vi "Normal Random.vi"(6 "seed":i32=-1, 7 "reset":bool, 9 "std":dbl=1.0, 10 "mean":dbl, 11 "samples":i32=128) -> (0 "error":i32, 3 "normal random data":dbl[](array[numeric]))   [LabVIEW 2024, in "NI_Gmath.lvlib"]
doc: "<p>Generates random values from a variate X, where X describes the selected distribution type. You must <a href=\"nihelplauncher://docs/csh?context=lvcore_lvhowto_selectingdefaultinstpolyvi\">manually select the polymorphic instance</a> to use.</p>"
uses:
  NI_Gmath.lvlib
  NI_AALBase.lvlib
panel:
  # "Normal Random"
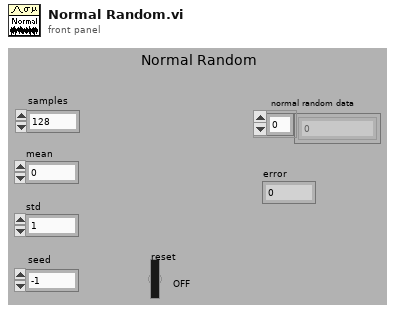
[diagram p1: front panel]
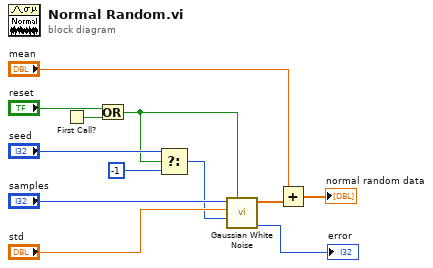
[diagram p0: block diagram]
diagram:
  n1 = First Call?() -> (First Call?: T/F=w12:bool)
  n2 = Or(x="reset", y=w12) -> (x .or. y?=w1:bool)
  n3 = Select(t="seed", s=w1, f=-1) -> (s? t:f=w3:i32)
  n4 = call "Gaussian White Noise.vi"("initialize?"=w1, "seed"=w3, "standard deviation"="std", "samples"="samples") -> ("error"=→"error":i32, "Gaussian noise pattern"=w8:dbl[])  [unwired: 6 in]
  n5 = Add(x="mean", y=w8) -> (x+y=→"normal random data":dbl[])
